vi "Recursion Got Nodes.vi"(8 "error in (no error)":errorcluster, 11 "Node Ptr":T1 format="%.0x") -> (0 "error out":errorcluster, 2 "Array":T1[](array[typedef]) format="%.0x", 3 "Node Ptr":T1 format="%.0x")   [LabVIEW 2023, in "Protection and Counter Support System Explorer.lvlib"]
uses:
  Protection and Counter Support System Explorer.lvlib
  <vilib>/NI VeriStand/Custom Device API/Custom Device Item Ref.ctl
  <vilib>/NI VeriStand/Custom Device API/Custom Device API.lvlib
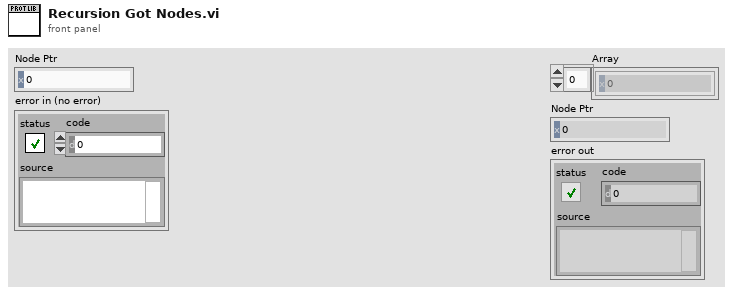
[diagram p1: front panel]
types:
  T1 = typedef "Custom Device API.lvlib/Custom Device Item Ref.ctl" = u64
  T2 = typedef "Custom Device API.lvlib/Custom Device Item Info.ctl" = cluster{"Name":string, "Is Channel":bool, "GUID":string, "Is Waveform":bool}
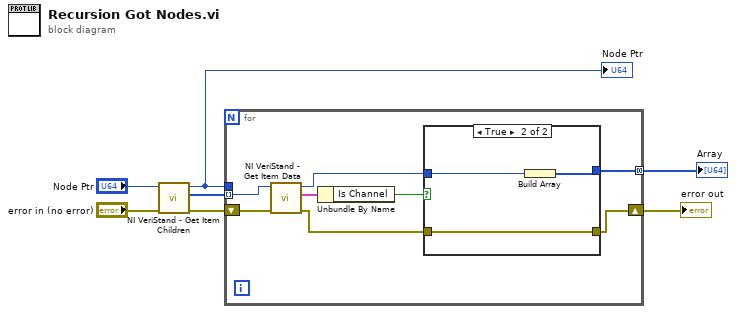
[diagram p0: block diagram]
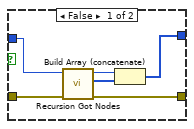
[diagram p2: hidden frame]
diagram:
  n1 = call <vilib>:"NI VeriStand - Get Item Children.vi"("error in (no error)"="error in (no error)", "Item Ref in"="Node Ptr") -> ("error out"=w4:errorcluster, "Child Refs"=w5:T1[], "Item Ref out"=w2:T1)  [unwired: 6 in, 1 out]
  "Node Ptr" <- w2
  n2 = for {
    tunnel: w2 -> [_]
    tunnel: w5 -> [w13] mode=indexing
    tunnel: [w11] -> w3 mode=concatenating
    shift-right: [w8] -> w1
    shift-left: w4 -> [w15]
    n3 = call <vilib>:"NI VeriStand - Get Item Data.vi"("error in (no error)"=w15, "Item Ref in"=w13) -> ("error out"=w9:errorcluster, "Item Info"=w14:T2, "Item Ref out"=w10:T1)  [unwired: 6 in, 1 out]
    n4 = Unbundle By Name(w14) -> ("Is Channel"=w12:bool)
    n5 = case shown="True" w12 {
      tunnel: [w20 w23] -> w11
      tunnel: w10 -> [w19 w24]
      tunnel: w9 -> [w17 w22]
      tunnel: [w16 w22] -> w8
      frame False {
        n6 = call "Recursion Got Nodes.vi"("error in (no error)"=w17, "Node Ptr"=w19) -> ("error out"=w16:errorcluster, "Array"=w21:T1[], "Node Ptr"=w18:T1)  [unwired: 7 in]
        n7 = Build Array (concatenate)(w18, w21) -> (w20:T1[])
      }
      frame True {
        n8 = Build Array(w24) -> (w23:T1[])
      }
    }
  }
  "Array" <- w3
  "error out" <- w1
